vi "RPC General Poll Response.vi"(8 "error in (no error)":errorcluster, 11 "BLE address in":string) -> (0 "error out":errorcluster, 1 "response":u8[](array[numeric]), 2 "polled":bool, 3 "BLE address out":string)   [LabVIEW 2017]
uses:
  nimble_sensor.dll
  <vilib>/addons/Bluetooth Sensing/Bluetooth Sensing.lvlib
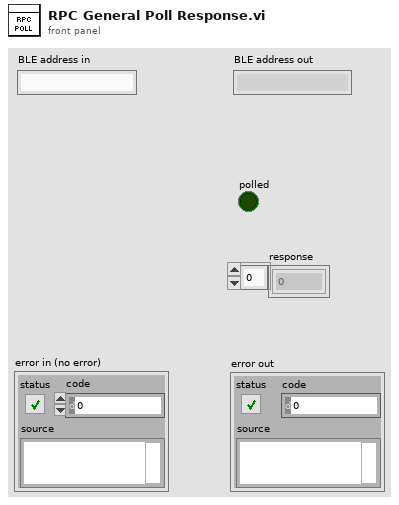
[diagram p1: front panel]
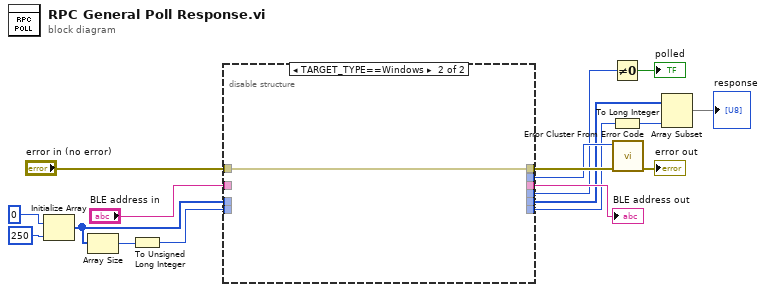
[diagram p0: block diagram]
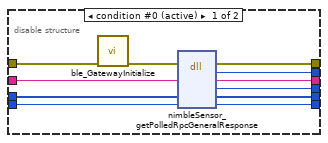
[diagram p2: hidden frame]
diagram:
  n1 = Initialize Array(u8 0, 250 ("dimension size")) -> (w9:u8[])
  n2 = Array Size(array=w9) -> (size(s)=w12:i32)
  n3 = To Unsigned Long Integer(number=w12) -> (unsigned 32bit integer=w2:u32)
  n4 = disable-structure shown="TARGET_TYPE==Windows" {
    disable-tunnel: "BLE address in" -> [w28 _]
    disable-tunnel: [w27 _] -> w16
    disable-tunnel: [w26 w29] -> w14
    disable-tunnel: [w25 _] -> w13
    disable-tunnel: w9 -> [w24 _]
    disable-tunnel: [w23 _] -> w8
    disable-tunnel: [w22 _] -> w6
    disable-tunnel: [w21 _] -> w5
    disable-tunnel: "error in (no error)" -> [w20 w29]
    disable-tunnel: w2 -> [w18 _]
    frame condition #0 (active) {
      n5 = call <vilib>:"ble_GatewayInitialize.vi"("error in (no error)"=w20) -> ("error out"=w19:errorcluster)  [unwired: 10 in]
      n6 = dll-call lib="nimble_sensor.*" fn="nimbleSensor_getPolledRpcGeneralResponse"(error in=w19, "address"=w28, "payload"=w24, "size"=w18) -> (error out=w26:errorcluster, "return type"=w25:i32, "address"=w27:string, "polled"=w23:u8, "payload"=w22:u8[], "size"=w21:u32)  [unwired: 3 in, 1 out]
    }
    frame condition #1 {
    }
  }
  "BLE address out" <- w16
  n7 = Not Equal To 0?(x=w8) -> (x != 0?=→"polled":bool)
  n8 = To Long Integer(number=w5) -> (32bit integer=w1:i32)
  n9 = call <vilib>:"Error Cluster From Error Code.vi"("error in (no error)"=w14, "error code (0)"=w13) -> ("error out"=→"error out":errorcluster)  [unwired: 7 in]
  n10 = Array Subset(array=w6, length=w1) -> (→"response":u8[])  [unwired: 1 in]
